vi "CMD_CHOICEPOPUP.vi"(8 "error in (no error)":errorcluster, 10 "Arguments":string[](array[string]), 11 "gScript Interpreter in":refnum<class "gScript Interpreter.lvclass">) -> (0 "error out":errorcluster, 3 "gScript Interpreter out":refnum<class "gScript Interpreter.lvclass">)   [LabVIEW 2017, in "gScript Interpreter.lvclass"]
uses:
  gScript Interpreter.lvclass
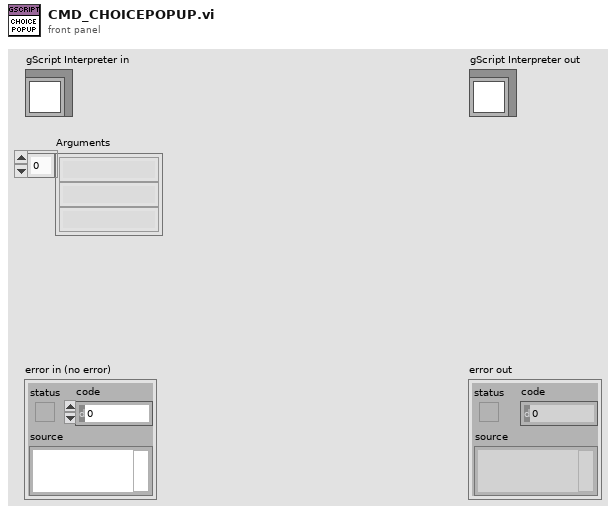
[diagram p1: front panel]
types:
  T1 = typedef "Memory Cell.ctl" = cluster{"type":T2, "x":dbl, "y":dbl, "z":dbl, "w":dbl}
  T2 = typedef "Memory Cell Type Enum.ctl" = enum16{"integer", "float", "vector", "rotation"}
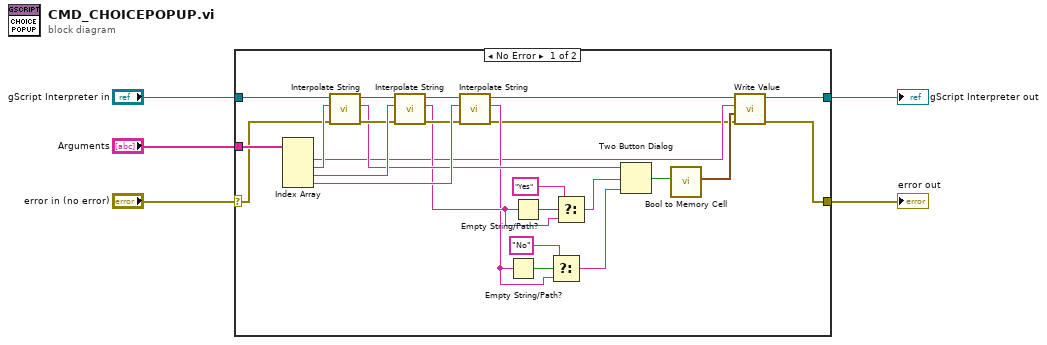
[diagram p0: block diagram]
diagram:
  n1 = case shown="No Error" "error in (no error)" {
    selector: "error in (no error)" -> [w18 w33]
    tunnel: [w7 w33] -> w4
    tunnel: [w6 w32] -> w2
    tunnel: "gScript Interpreter in" -> [w24 w32]
    tunnel: "Arguments" -> [w31 _]
    frame No Error {
      n2 = Index Array(array=w31) -> (element #1=w9:string, element #2=w21:string, element #3=w20:string, element #4=w19:string)  [unwired: 4 in]
      n3 = call-dynamic "Interpolate String.vi"("error in (no error)"=w18, "Input String"=w21, "gScript Interpreter in"=w24) -> ("error out"=w17:errorcluster, "Output String"=w15:string, "gScript Interpreter out"=w23:refnum<class "gScript Interpreter.lvclass">)  [unwired: 6 in]
      n4 = call-dynamic "Interpolate String.vi"("error in (no error)"=w17, "Input String"=w20, "gScript Interpreter in"=w23) -> ("error out"=w16:errorcluster, "Output String"=w14:string, "gScript Interpreter out"=w22:refnum<class "gScript Interpreter.lvclass">)  [unwired: 6 in]
      n5 = call-dynamic "Interpolate String.vi"("error in (no error)"=w16, "Input String"=w19, "gScript Interpreter in"=w22) -> ("error out"=w8:errorcluster, "Output String"=w13:string, "gScript Interpreter out"=w12:refnum<class "gScript Interpreter.lvclass">)  [unwired: 6 in]
      n6 = Empty String/Path?(string/path=w13) -> (empty?=w28:bool)
      n7 = Empty String/Path?(string/path=w14) -> (empty?=w30:bool)
      n8 = Select(t="No", s=w28, f=w13) -> (s? t:f=w25:string)
      n9 = Select(t="Yes", s=w30, f=w14) -> (s? t:f=w26:string)
      n10 = Two Button Dialog(message=w15, 1:w25, 2:w26) -> (T button?=w11:bool)
      n11 = call "Bool to Memory Cell.vi"("Boolean in"=w11) -> ("Memory Cell"=w10:T1)  [unwired: 10 in]
      n12 = call-dynamic "Write Value.vi"("error in (no error)"=w8, "Value"=w10, "Address"=w9, "gScript Interpreter in"=w12) -> ("error out"=w7:errorcluster, "gScript Interpreter out"=w6:refnum<class "gScript Interpreter.lvclass">)  [unwired: 6 in]
    }
    frame Error {
    }
  }
  "error out" <- w4
  "gScript Interpreter out" <- w2
